vi "applyDM_and_trigEMCCD.vi"(5 "Absolute Positions":T1, 7 "WavefrontCorrector in":refnum<class "WavefrontCorrector.lvclass">, 8 "error in (no error)":errorcluster, 9 "Trig Num":i32, 10 "exp and readout time (ms)":dbl, 11 "EMCCD trigger port":tag="Dev1/port0/line0") -> (0 "error out":errorcluster, 3 "WavefrontCorrector out":refnum<class "WavefrontCorrector.lvclass">)   [LabVIEW 2018]
uses:
  <userlib>/WaveKit.lib/Classes/WavefrontCorrector/WavefrontCorrector.lvclass
  <userlib>/WaveKit.lib/Controls/Wavefront Corrector Position.ctl
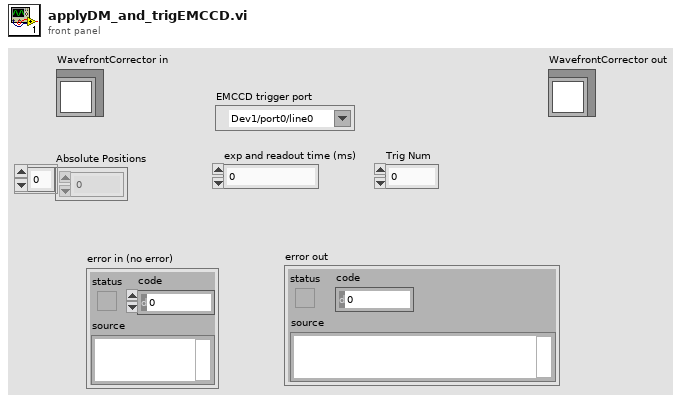
[diagram p1: front panel]
types:
  T1 = typedef "Wavefront Corrector Position.ctl" = sgl[]
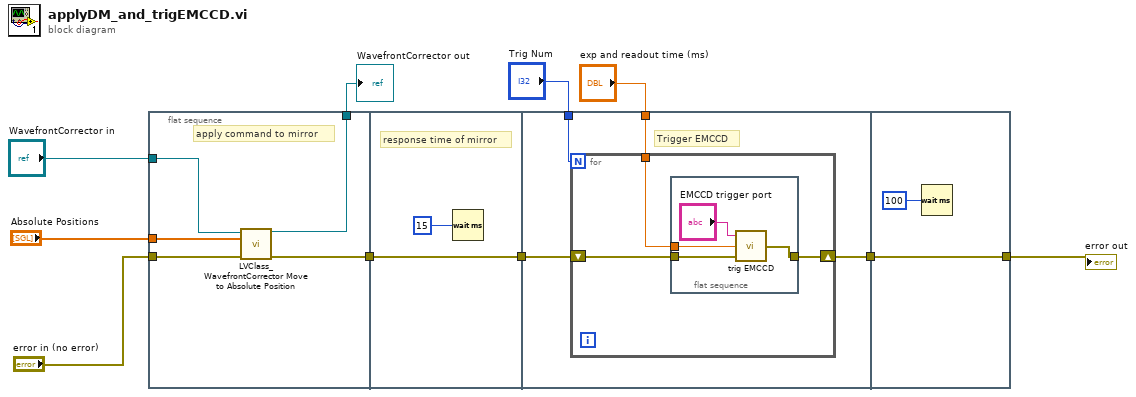
[diagram p0: block diagram]
diagram:
  n1 = flat-sequence {
    tunnel: [w15] -> w9
    tunnel: "WavefrontCorrector in" -> [w14]
    tunnel: "error in (no error)" -> [w13]
    tunnel: [w12] -> w4
    tunnel: "Absolute Positions" -> [w11]
    tunnel: [w16] -> w10
    tunnel: w9 -> [w16]
    tunnel: w10 -> [w21]
    tunnel: "exp and readout time (ms)" -> [w19]
    tunnel: "Trig Num" -> [w18]
    tunnel: [w20] -> w1
    tunnel: [w30] -> w6
    tunnel: w1 -> [w30]
    frame #0 {
      # "apply command to mirror"
      n2 = call <userlib>:"LVClass_WavefrontCorrector Move to Absolute Position.vi"("WavefrontCorrector in"=w14, "Absolute Positions"=w11, "error in (no error)"=w13) -> ("WavefrontCorrector out"=w12:refnum<class "WavefrontCorrector.lvclass">, "error out"=w15:errorcluster)  [unwired: 11 in]
    }
    frame #1 {
      # "response time of mirror"
      n3 = Wait (ms)(milliseconds to wait=15) -> ()  [unwired: 1 out]
    }
    frame #2 {
      # "Trigger EMCCD"
      n4 = for {
        N: w18 -> [_]
        shift-right: [w23] -> w20
        shift-left: w21 -> [w24]
        tunnel: w19 -> [w22]
        n5 = flat-sequence {
          tunnel: w24 -> [w27]
          tunnel: w22 -> [w25]
          tunnel: [w26] -> w23
          frame #0 {
            n6 = call "trig EMCCD.vi"("error in (no error)"=w27, "camera time"=w25, "lines"="EMCCD trigger port") -> ("error out"=w26:errorcluster)
          }
        }
      }
    }
    frame #3 {
      n7 = Wait (ms)(milliseconds to wait=100) -> ()  [unwired: 1 out]
    }
  }
  "error out" <- w6
  "WavefrontCorrector out" <- w4
